vi "Comms Loop.vi"(8 "error in (no error)":errorcluster, 11 "FormulaG App in":refnum<class "FormulaG App.lvclass">) -> (0 "error out":errorcluster)   [LabVIEW 2020, in "FormulaG.lvlib" / "FormulaG App.lvclass"]
uses:
  FormulaG App.lvclass
  FormulaG App.lvclass/FormulaG App.ctl
  State Update.ctl
  FormulaG-Common/Car State.ctl
  FormulaG-Common/Ranges.ctl
  FormulaG-Common/Car Info.ctl
  FormulaG-Common/Car Control.ctl
  FormulaG API/FormulaG API.lvclass
  FormulaG-Common/FormulaG-Common.lvlib
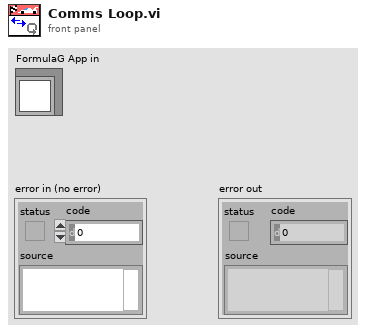
[diagram p1: front panel]
types:
  T1 = typedef "FormulaG-Common.lvlib/Control VI.ctl" = refnum<vi>
  T2 = typedef "FormulaG.lvlib/FormulaG App.lvclass/State Update.ctl" = cluster{"Car State":T3, "Car Control":T6}
  T3 = typedef "FormulaG-Common.lvlib/Car State.ctl" = cluster{"Ranges":T4, "Car Info":T5, "Current Lap":dbl, "Last Lap":dbl}
  T4 = typedef "FormulaG-Common.lvlib/Ranges.ctl" = cluster{"Front":sgl[], "Rear":sgl[]}
  T5 = typedef "FormulaG-Common.lvlib/Car Info.ctl" = cluster{"Speed":sgl, "X":sgl, "Y":sgl, "Heading":sgl}
  T6 = typedef "FormulaG-Common.lvlib/Car Control.ctl" = cluster{"Steering (-1 to 1)":sgl, "Throttle (0 to 1)":sgl}
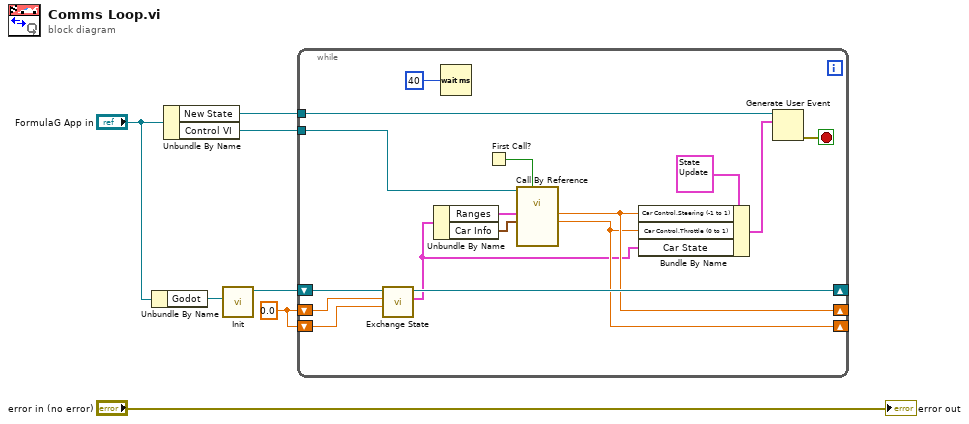
[diagram p0: block diagram]
diagram:
  w1 = sgl 0.0 ("Steering (-1 to 1)")
  n1 = Unbundle By Name("FormulaG App in") -> ("Godot"=w6:refnum<class "GodotServer.lvclass">)
  n2 = Unbundle By Name("FormulaG App in") -> ("New State"=w2:refnum<user-event>, "Control VI"=w3:T1)
  n3 = call "Init.vi"("Godot"=w6) -> ("FormulaG API out"=w5:refnum<class "FormulaG API.lvclass">)  [unwired: 9 in, 1 out]
  n4 = while {
    shift-right: [w18] -> _
    shift-left: w5 -> [w22]
    tunnel: w3 -> [w21]
    shift-right: [w15] -> _
    shift-left: w1 -> [w17]
    shift-right: [w14] -> _
    shift-left: w1 -> [w16]
    tunnel: w2 -> [w12]
    stop <- w10 stop-if-true
    n5 = call "Exchange State.vi"("Throttle"=w16, "Steering"=w17, "FormulaG API in"=w22) -> ("Car State"=w13:T3, "FormulaG API out"=w18:refnum<class "FormulaG API.lvclass">)  [unwired: 6 in, 1 out]
    n6 = Unbundle By Name(w13) -> ("Ranges"=w20:T4, "Car Info"=w19:T5)
    n7 = Wait (ms)(milliseconds to wait=u32 40) -> ()  [unwired: 1 out]
    n8 = First Call?() -> (First Call?: T/F=w8:bool)
    n9 = call-by-ref "?"(reference=w21, "Reset"=w8, "Car Info"=w19, "Ranges"=w20) -> ("Throttle (0 to 1)"=w14:sgl, "Steering (-1 to 1)"=w15:sgl)  [unwired: 8 in, 2 out]
    n10 = Bundle By Name(cluster=T2 {"Car State"={"Ranges"={"Front"=[], "Rear"=[]}, "Car Info"={"Speed"=0.0, "X"=0.0, "Y"=0.0, "Heading"=0.0}, "Current Lap"=0.0, "Last Lap"=0.0}, "Car Control"={"Steering (-1 to 1)"=0.0, "Throttle (0 to 1)"=0.0}} ("State Update"), "Car Control.Steering (-1 to 1)"=w15, "Car Control.Throttle (0 to 1)"=w14, "Car State"=w13) -> (w11:T2)
    n11 = Generate User Event(user event=w12, event data cluster=w11) -> (error out=w10:errorcluster)  [unwired: 2 in, 1 out]
  }
  "error out" <- "error in (no error)"
